vi "RPN Arithmetic Solver.vi"(0 "Solver Input (Postfix) Data":T1, 1 "error in (no error)":errorcluster) -> (2 "Answer (numeric)":dbl, 3 "Answer (string)":string, 5 "error out":errorcluster)   [LabVIEW 2020]
uses:
  <vilib>/Utility/error.llb/Error Cluster From Error Code.vi
  <vilib>/ErrorRing/Error Ring.xnode
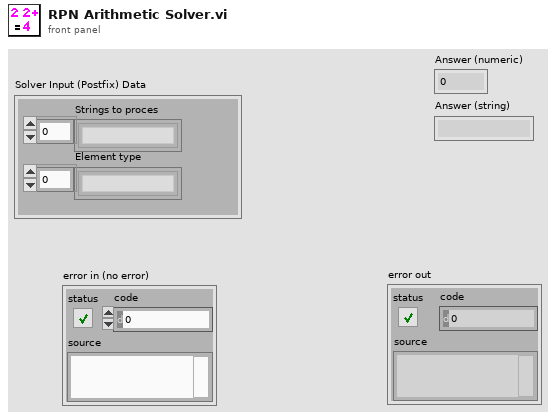
[diagram p1: front panel]
types:
  T1 = cluster{"Strings to proces":string[], "Element type":string[]}
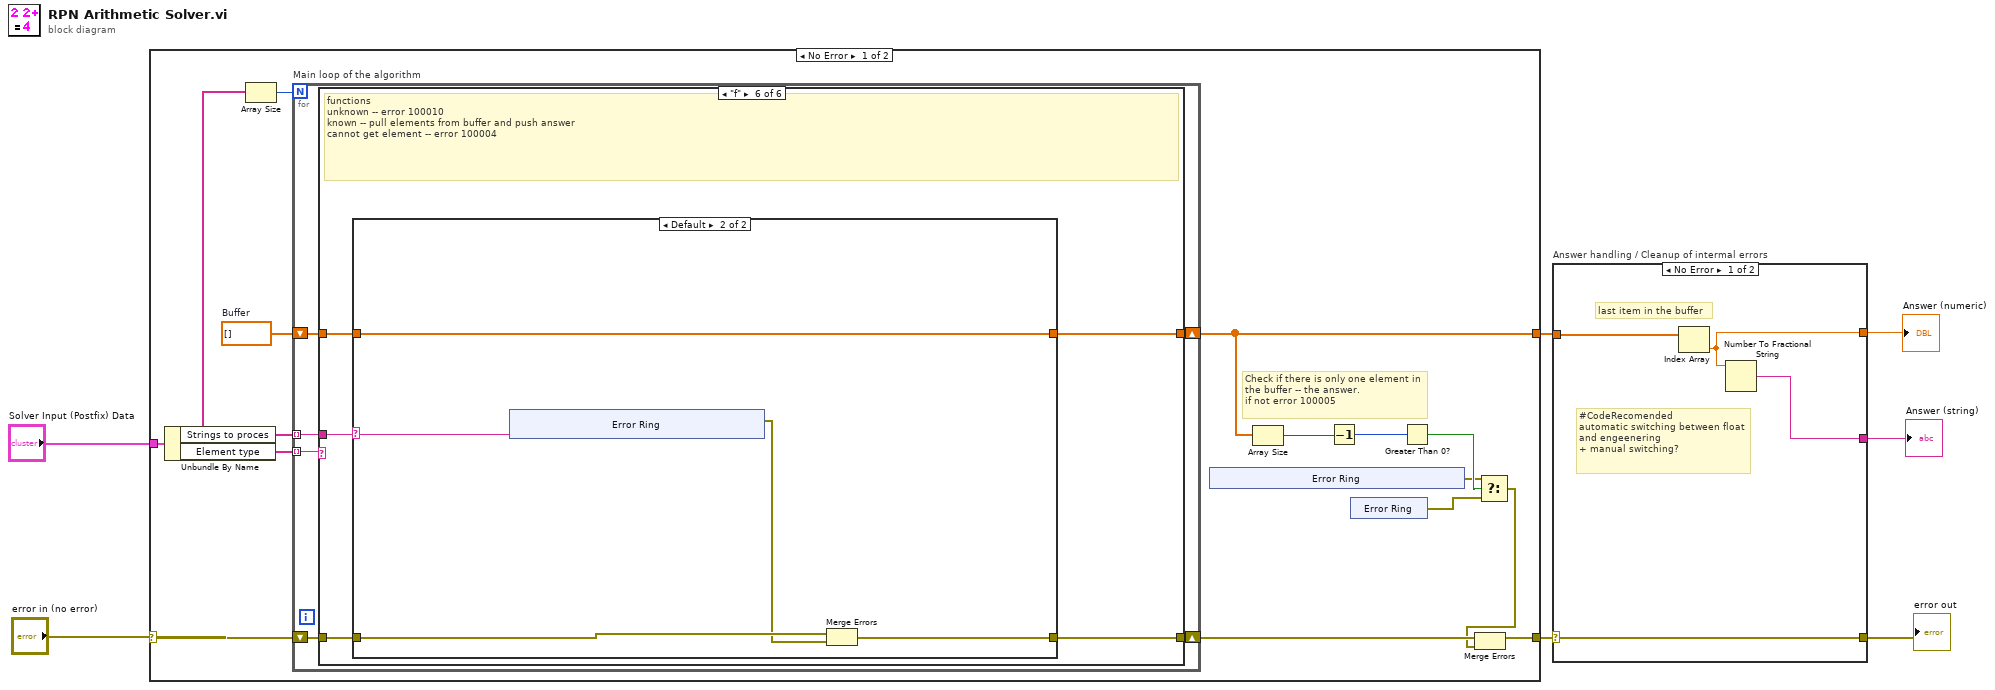
[diagram p0: block diagram]
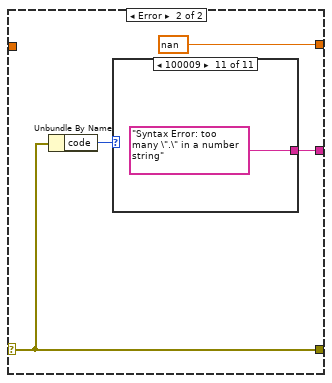
[diagram p2: hidden frame]
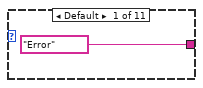
[diagram p3: hidden frame]
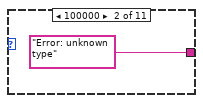
[diagram p4: hidden frame]
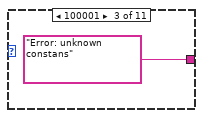
[diagram p5: hidden frame]
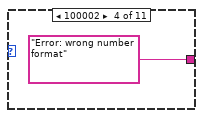
[diagram p6: hidden frame]
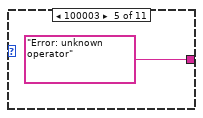
[diagram p7: hidden frame]
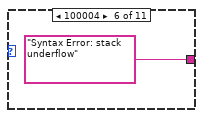
[diagram p8: hidden frame]
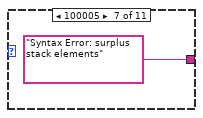
[diagram p9: hidden frame]
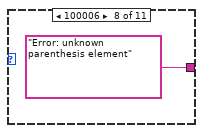
[diagram p10: hidden frame]
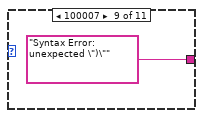
[diagram p11: hidden frame]
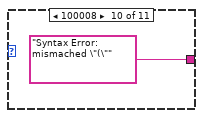
[diagram p12: hidden frame]
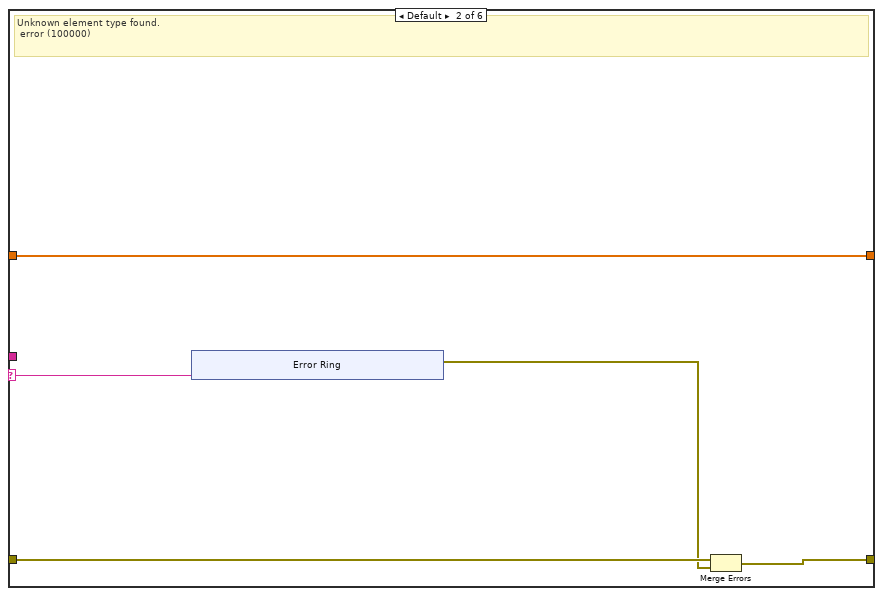
[diagram p14: hidden frame]
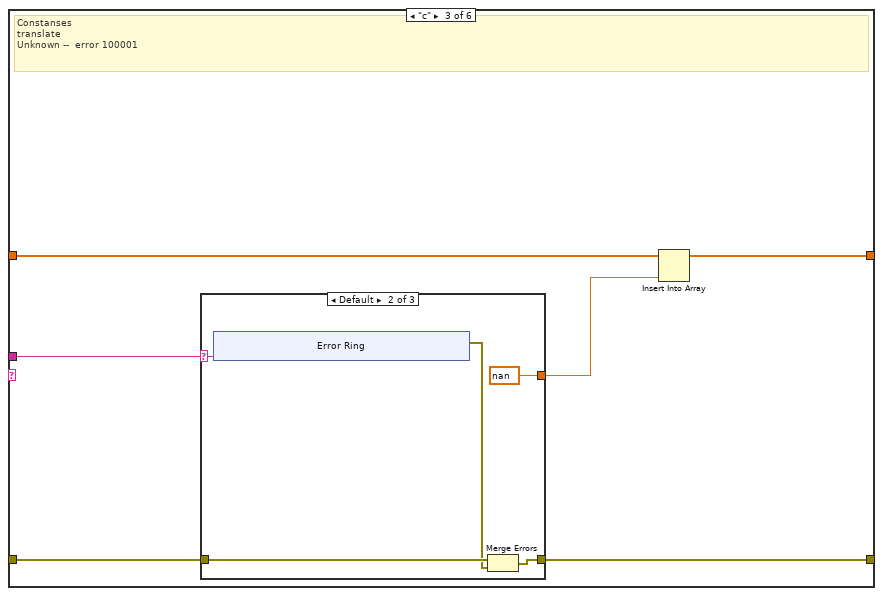
[diagram p15: hidden frame]
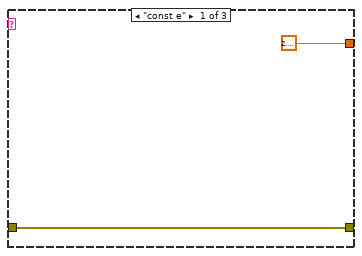
[diagram p16: hidden frame]
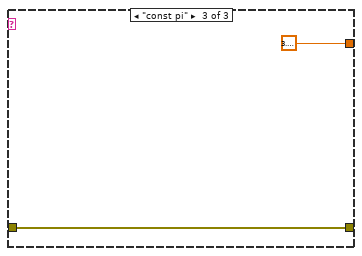
[diagram p17: hidden frame]
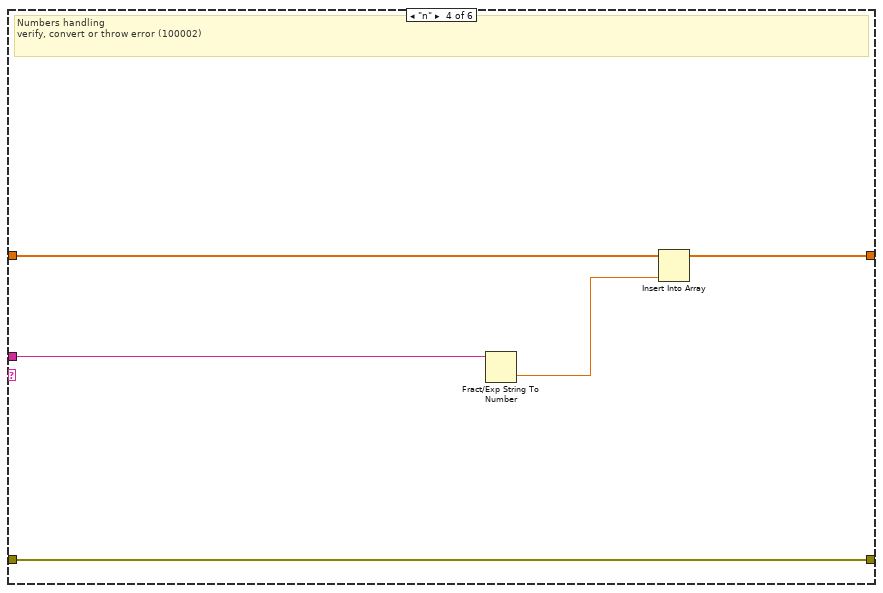
[diagram p18: hidden frame]
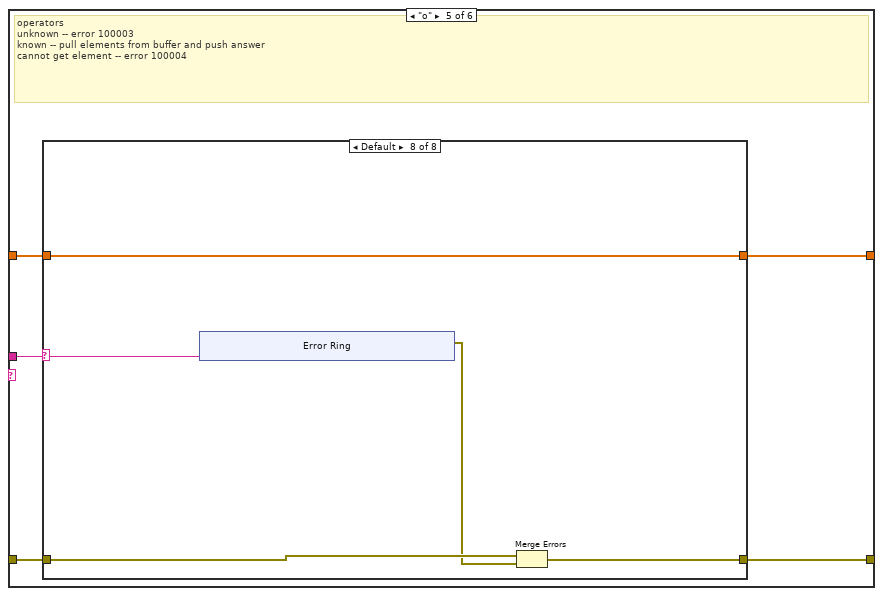
[diagram p19: hidden frame]
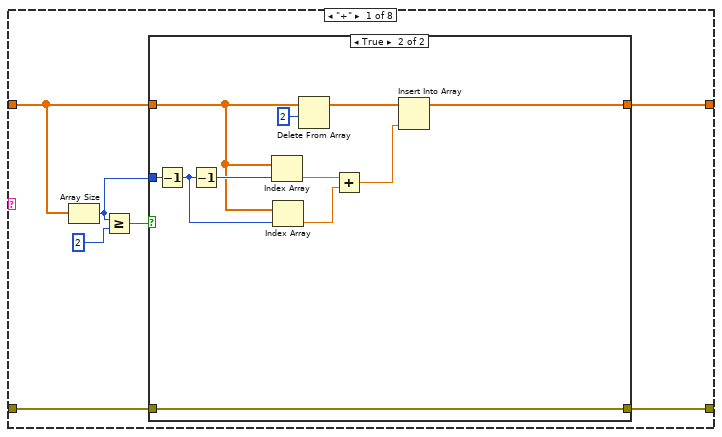
[diagram p20: hidden frame]
diagram:
  n1 = case shown="No Error" "error in (no error)" {
    selector: "error in (no error)" -> [w22 w318]
    tunnel: [w13 w318] -> w4
    tunnel: "Solver Input (Postfix) Data" -> [w20 _]
    tunnel: [w12 w317] -> w5
    frame No Error {
      w21 = dbl[] []  # Buffer
      # "Check if there is only one element in the buffer -- the answer.\nif not error 100005"
      n2 = Unbundle By Name(w20) -> ("Strings to proces"=w17:string[], "Element type"=w19:string[])
      n3 = Array Size(array=w17) -> (size(s)=w18:i32)
      n4 = for "Main loop of the algorithm" {
        N: w18 -> [_]
        shift-right: [w29] -> w14
        shift-left: w22 -> [w30]
        shift-right: [w31] -> w12
        shift-left: w21 -> [w32]
        tunnel: w17 -> [w33] mode=indexing
        tunnel: w19 -> [w34] mode=indexing
        n5 = case shown="\"f\"" w34 {
          selector: w34 -> [_ w40 _ _ _ _]
          tunnel: w33 -> [_ _ w52 w72 w74 w277]
          tunnel: w32 -> [w36 w41 w54 w71 w76 w279]
          tunnel: [w36 w41 w53 w70 w75 w278] -> w31
          tunnel: w30 -> [w35 w38 w50 w73 w78 w281]
          tunnel: [w35 w39 w49 w73 w77 w280] -> w29
          frame "" {
            # "Blanks\nignore"
          }
          frame Default {
            # "Unknown element type found.\n error (100000)"
            n6 = xnode "Error Ring"("parameter 0"=w40) -> ("error out"=w37:errorcluster)
            n7 = Merge Errors(w38, w37) -> (w39:errorcluster)
          }
          frame "c" {
            # "Constanses\ntranslate\nUnknown --  error 100001"
            n8 = case shown="Default" w52 {
              selector: w52 -> [_ w60 _]
              tunnel: [2.718281828459045 nan 3.141592653589793] -> w51
              tunnel: w50 -> [w55 w58 w67]
              tunnel: [w55 w59 w67] -> w49
              frame "const e" {
              }
              frame Default {
                n9 = xnode "Error Ring"("parameter 0"=w60) -> ("error out"=w57:errorcluster)
                n10 = Merge Errors(w58, w57) -> (w59:errorcluster)
              }
              frame "const pi" {
              }
            }
            n11 = Insert Into Array(array=w54, new element=w51) -> (w53:dbl[])  [unwired: 1 in]
          }
          frame "n" {
            # "Numbers handling\nverify, convert or throw error (100002)"
            n12 = Fract/Exp String To Number(string=w72) -> (number=w69:dbl)  [unwired: 3 in, 1 out]
            n13 = Insert Into Array(array=w71, new element=w69) -> (w70:dbl[])  [unwired: 1 in]
          }
          frame "o" {
            # "operators\nunknown -- error 100003\nknown -- pull elements from buffer and push answer \ncannot get element -- error 100004"
            n14 = case shown="Default" w74 {
              selector: w74 -> [_ _ _ _ _ _ _ w270]
              tunnel: w78 -> [w84 w111 w138 w163 w190 w217 w244 w269]
              tunnel: [w85 w112 w139 w164 w191 w218 w245 w268] -> w77
              tunnel: w76 -> [w83 w110 w137 w162 w189 w216 w243 w271]
              tunnel: [w82 w109 w136 w161 w188 w215 w242 w271] -> w75
              frame "+" {
                n15 = Array Size(array=w83) -> (size(s)=w79:i32)
                n16 = Greater Or Equal?(x=w79, y=2) -> (x >= y?=w81:bool)
                n17 = case shown="True" w81 {
                  tunnel: [w89 w105] -> w85
                  tunnel: w84 -> [w88 w105]
                  tunnel: w83 -> [_ w101]
                  tunnel: [dbl[] [] ("Buffer") w99] -> w82
                  tunnel: w79 -> [_ w104]
                  frame False {
                    n18 = xnode "Error Ring"() -> ("error out"=w87:errorcluster)
                    n19 = Merge Errors(w88, w87) -> (w89:errorcluster)
                  }
                  frame True {
                    n20 = Decrement(x=w104) -> (x-1=w103:i32)
                    n21 = Decrement(x=w103) -> (x-1=w102:i32)
                    n22 = Index Array(array=w101, index=w102) -> (element=w95:dbl)
                    n23 = Index Array(array=w101, index=w103) -> (element=w96:dbl)
                    n24 = Delete From Array(array=w101, length=2) -> (array with subset deleted=w100:dbl[])  [unwired: 1 in, 1 out]
                    n25 = Add(x=w95, y=w96) -> (x+y=w98:dbl)
                    n26 = Insert Into Array(array=w100, new element=w98) -> (w99:dbl[])  [unwired: 1 in]
                  }
                }
              }
              frame "-" {
                n27 = Array Size(array=w110) -> (size(s)=w106:i32)
                n28 = Greater Or Equal?(x=w106, y=2) -> (x >= y?=w108:bool)
                n29 = case shown="True" w108 {
                  tunnel: [w116 w132] -> w112
                  tunnel: w111 -> [w115 w132]
                  tunnel: w110 -> [_ w128]
                  tunnel: [dbl[] [] ("Buffer") w126] -> w109
                  tunnel: w106 -> [_ w131]
                  frame False {
                    n30 = xnode "Error Ring"() -> ("error out"=w114:errorcluster)
                    n31 = Merge Errors(w115, w114) -> (w116:errorcluster)
                  }
                  frame True {
                    n32 = Decrement(x=w131) -> (x-1=w130:i32)
                    n33 = Decrement(x=w130) -> (x-1=w129:i32)
                    n34 = Index Array(array=w128, index=w129) -> (element=w123:dbl)
                    n35 = Index Array(array=w128, index=w130) -> (element=w122:dbl)
                    n36 = Delete From Array(array=w128, length=2) -> (array with subset deleted=w127:dbl[])  [unwired: 1 in, 1 out]
                    n37 = Subtract(x=w123, y=w122) -> (x-y=w125:dbl)
                    n38 = Insert Into Array(array=w127, new element=w125) -> (w126:dbl[])  [unwired: 1 in]
                  }
                }
              }
              frame "NEG" {
                n39 = Array Size(array=w137) -> (size(s)=w133:i32)
                n40 = Greater Or Equal?(x=w133, y=1) -> (x >= y?=w135:bool)
                n41 = case shown="True" w135 {
                  tunnel: [w143 w157] -> w139
                  tunnel: w138 -> [w142 w157]
                  tunnel: w137 -> [_ w155]
                  tunnel: [dbl[] [] ("Buffer") w153] -> w136
                  tunnel: w133 -> [_ w156]
                  frame False {
                    n42 = xnode "Error Ring"() -> ("error out"=w141:errorcluster)
                    n43 = Merge Errors(w142, w141) -> (w143:errorcluster)
                  }
                  frame True {
                    n44 = Decrement(x=w156) -> (x-1=w149:i32)
                    n45 = Index Array(array=w155, index=w149) -> (element=w150:dbl)
                    n46 = Delete From Array(array=w155, length=1) -> (array with subset deleted=w154:dbl[])  [unwired: 1 in, 1 out]
                    n47 = Negate(x=w150) -> (-x=w152:dbl)
                    n48 = Insert Into Array(array=w154, new element=w152) -> (w153:dbl[])  [unwired: 1 in]
                  }
                }
              }
              frame "*" {
                n49 = Array Size(array=w162) -> (size(s)=w158:i32)
                n50 = Greater Or Equal?(x=w158, y=2) -> (x >= y?=w160:bool)
                n51 = case shown="True" w160 {
                  tunnel: [w168 w184] -> w164
                  tunnel: w163 -> [w167 w184]
                  tunnel: w162 -> [_ w180]
                  tunnel: [dbl[] [] ("Buffer") w178] -> w161
                  tunnel: w158 -> [_ w183]
                  frame False {
                    n52 = xnode "Error Ring"() -> ("error out"=w166:errorcluster)
                    n53 = Merge Errors(w167, w166) -> (w168:errorcluster)
                  }
                  frame True {
                    n54 = Decrement(x=w183) -> (x-1=w182:i32)
                    n55 = Decrement(x=w182) -> (x-1=w181:i32)
                    n56 = Index Array(array=w180, index=w181) -> (element=w175:dbl)
                    n57 = Index Array(array=w180, index=w182) -> (element=w174:dbl)
                    n58 = Delete From Array(array=w180, length=2) -> (array with subset deleted=w179:dbl[])  [unwired: 1 in, 1 out]
                    n59 = Multiply(x=w175, y=w174) -> (x*y=w177:dbl)
                    n60 = Insert Into Array(array=w179, new element=w177) -> (w178:dbl[])  [unwired: 1 in]
                  }
                }
              }
              frame "/" {
                n61 = Array Size(array=w189) -> (size(s)=w185:i32)
                n62 = Greater Or Equal?(x=w185, y=2) -> (x >= y?=w187:bool)
                n63 = case shown="True" w187 {
                  tunnel: [w195 w211] -> w191
                  tunnel: w190 -> [w194 w211]
                  tunnel: w189 -> [_ w207]
                  tunnel: [dbl[] [] ("Buffer") w205] -> w188
                  tunnel: w185 -> [_ w210]
                  frame False {
                    n64 = xnode "Error Ring"() -> ("error out"=w193:errorcluster)
                    n65 = Merge Errors(w194, w193) -> (w195:errorcluster)
                  }
                  frame True {
                    n66 = Decrement(x=w210) -> (x-1=w209:i32)
                    n67 = Decrement(x=w209) -> (x-1=w208:i32)
                    n68 = Index Array(array=w207, index=w208) -> (element=w202:dbl)
                    n69 = Index Array(array=w207, index=w209) -> (element=w201:dbl)
                    n70 = Delete From Array(array=w207, length=2) -> (array with subset deleted=w206:dbl[])  [unwired: 1 in, 1 out]
                    n71 = Divide(x=w202, y=w201) -> (x/y=w204:dbl)
                    n72 = Insert Into Array(array=w206, new element=w204) -> (w205:dbl[])  [unwired: 1 in]
                  }
                }
              }
              frame "^" {
                n73 = Array Size(array=w216) -> (size(s)=w212:i32)
                n74 = Greater Or Equal?(x=w212, y=2) -> (x >= y?=w214:bool)
                n75 = case shown="True" w214 {
                  tunnel: [w222 w238] -> w218
                  tunnel: w217 -> [w221 w238]
                  tunnel: w216 -> [_ w234]
                  tunnel: [dbl[] [] ("Buffer") w232] -> w215
                  tunnel: w212 -> [_ w237]
                  frame False {
                    n76 = xnode "Error Ring"() -> ("error out"=w220:errorcluster)
                    n77 = Merge Errors(w221, w220) -> (w222:errorcluster)
                  }
                  frame True {
                    n78 = Decrement(x=w237) -> (x-1=w236:i32)
                    n79 = Decrement(x=w236) -> (x-1=w235:i32)
                    n80 = Index Array(array=w234, index=w236) -> (element=w229:dbl)
                    n81 = Index Array(array=w234, index=w235) -> (element=w230:dbl)
                    n82 = Delete From Array(array=w234, length=2) -> (array with subset deleted=w233:dbl[])  [unwired: 1 in, 1 out]
                    n83 = Power Of X(1:w230, 2:w229) -> (0:w228:dbl)
                    n84 = Insert Into Array(array=w233, new element=w228) -> (w232:dbl[])  [unwired: 1 in]
                  }
                }
              }
              frame "E" {
                n85 = Array Size(array=w243) -> (size(s)=w239:i32)
                n86 = Greater Or Equal?(x=w239, y=2) -> (x >= y?=w241:bool)
                n87 = case shown="True" w241 {
                  tunnel: [w249 w266] -> w245
                  tunnel: w244 -> [w248 w266]
                  tunnel: w243 -> [_ w262]
                  tunnel: [dbl[] [] ("Buffer") w260] -> w242
                  tunnel: w239 -> [_ w265]
                  frame False {
                    n88 = xnode "Error Ring"() -> ("error out"=w247:errorcluster)
                    n89 = Merge Errors(w248, w247) -> (w249:errorcluster)
                  }
                  frame True {
                    n90 = Decrement(x=w265) -> (x-1=w264:i32)
                    n91 = Decrement(x=w264) -> (x-1=w263:i32)
                    n92 = Index Array(array=w262, index=w264) -> (element=w258:dbl)
                    n93 = Index Array(array=w262, index=w263) -> (element=w257:dbl)
                    n94 = Delete From Array(array=w262, length=2) -> (array with subset deleted=w261:dbl[])  [unwired: 1 in, 1 out]
                    n95 = Power Of 10(x=w258) -> (10^x=w256:dbl)
                    n96 = Multiply(x=w256, y=w257) -> (x*y=w255:dbl)
                    n97 = Insert Into Array(array=w261, new element=w255) -> (w260:dbl[])  [unwired: 1 in]
                  }
                }
              }
              frame Default {
                n98 = xnode "Error Ring"("parameter 0"=w270) -> ("error out"=w267:errorcluster)
                n99 = Merge Errors(w269, w267) -> (w268:errorcluster)
              }
            }
          }
          frame "f" {
            # "functions\nunknown -- error 100010\nknown -- pull elements from buffer and push answer \ncannot get element -- error 100004"
            n100 = case shown="Default" w277 {
              selector: w277 -> [_ w310]
              tunnel: w281 -> [w287 w309]
              tunnel: [w288 w308] -> w280
              tunnel: w279 -> [w286 w311]
              tunnel: [w285 w311] -> w278
              frame "sin" {
                n101 = Array Size(array=w286) -> (size(s)=w282:i32)
                n102 = Greater Or Equal?(x=w282, y=1) -> (x >= y?=w284:bool)
                n103 = case shown="True" w284 {
                  tunnel: [w292 w306] -> w288
                  tunnel: w287 -> [w291 w306]
                  tunnel: w286 -> [_ w304]
                  tunnel: [dbl[] [] ("Buffer") w302] -> w285
                  tunnel: w282 -> [_ w305]
                  frame False {
                    n104 = xnode "Error Ring"() -> ("error out"=w290:errorcluster)
                    n105 = Merge Errors(w291, w290) -> (w292:errorcluster)
                  }
                  frame True {
                    n106 = Decrement(x=w305) -> (x-1=w298:i32)
                    n107 = Index Array(array=w304, index=w298) -> (element=w299:dbl)
                    n108 = Delete From Array(array=w304, length=1) -> (array with subset deleted=w303:dbl[])  [unwired: 1 in, 1 out]
                    n109 = Sine(x=w299) -> (sin(x)=w301:dbl)
                    n110 = Insert Into Array(array=w303, new element=w301) -> (w302:dbl[])  [unwired: 1 in]
                  }
                }
              }
              frame Default {
                n111 = xnode "Error Ring"("parameter 0"=w310) -> ("error out"=w307:errorcluster)
                n112 = Merge Errors(w309, w307) -> (w308:errorcluster)
              }
            }
          }
        }
      }
      n113 = xnode "Error Ring"() -> ("error out"=w9:errorcluster)
      n114 = Array Size(array=w12) -> (size(s)=w16:i32)
      n115 = Decrement(x=w16) -> (x-1=w15:i32)
      n116 = xnode "Error Ring"() -> ("error out"=w8:errorcluster)
      n117 = Greater Than 0?(x=w15) -> (x > 0?=w11:bool)
      n118 = Select(t=w9, s=w11, f=w8) -> (s? t:f=w10:errorcluster)
      n119 = Merge Errors(w14, w10) -> (w13:errorcluster)
    }
    frame Error {
      w317 = dbl[] []  # Dummy
    }
  }
  n120 = case "Answer handling / Cleanup of intermal errors" shown="No Error" w4 {
    selector: w4 -> [w322 w323]
    tunnel: [w322 w323] -> w1
    tunnel: [w319 w325] -> w3
    tunnel: [w320 nan] -> w2
    tunnel: w5 -> [w321 _]
    frame No Error {
      # "last item in the buffer"
      # "#CodeRecomended\nautomatic switching between float and engeenering\n+ manual switching?"
      n121 = Index Array(array=w321) -> (element=w320:dbl)  [unwired: 1 in]
      n122 = Number To Fractional String(number=w320) -> (F-format string=w319:string)  [unwired: 3 in]
    }
    frame Error {
      n123 = Unbundle By Name(w323) -> ("code"=w326:i32)
      n124 = case shown="100009" w326 {
        tunnel: ["Error" "Error: unknown type" "Error: unknown constans" "Error: wrong number format" "Error: unknown operator" "Syntax Error: stack underflow" "Syntax Error: surplus stack elements" "Error: unknown parenthesis element" "Syntax Error: unexpected \")\"" "Syntax Error: mismached \"(\"" "Syntax Error: too many \".\" in a number string"] -> w325
        frame Default {
        }
        frame 100000 {
        }
        frame 100001 {
        }
        frame 100002 {
        }
        frame 100003 {
        }
        frame 100004 {
        }
        frame 100005 {
        }
        frame 100006 {
        }
        frame 100007 {
        }
        frame 100008 {
        }
        frame 100009 {
        }
      }
    }
  }
  "Answer (string)" <- w3
  "error out" <- w1
  "Answer (numeric)" <- w2
